vi "Escape JSON.vi"(11 "String in":string) -> (3 "String out":string)   [LabVIEW 2017, in "Front Panel Publisher.lvlib" / "String.lvclass"]
uses:
  String.lvclass
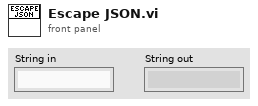
[diagram p1: front panel]
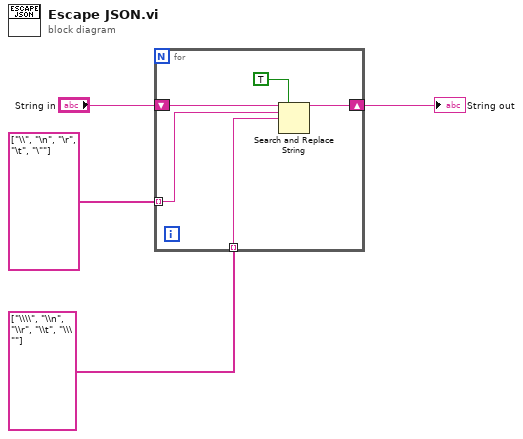
[diagram p0: block diagram]
diagram:
  n1 = for {
    shift-right: [w7] -> w3
    shift-left: "String in" -> [w8]
    tunnel: string[] ["\\", "\n", "\r", "\t", "\""] -> [w6] mode=indexing
    tunnel: string[] ["\\\\", "\\n", "\\r", "\\t", "\\\""] -> [w5] mode=indexing
    n2 = Search and Replace String(replace all?=TRUE ("replace all? (F)"), input string=w8, search string=w6, replace string=w5) -> (result string=w7:string)  [unwired: 4 in, 3 out]
  }
  "String out" <- w3
